vi "NXT_HINDBRAIN NXT Buttons To String.vi"(1 "_NXTButtonStates":bool[](array[boolean])) -> (0 "String":string)   [LabVIEW 2012, in "Tugboat.lvrbt"]
uses:
  Tugboat.lvrbt
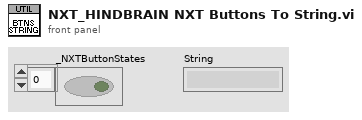
[diagram p1: front panel]
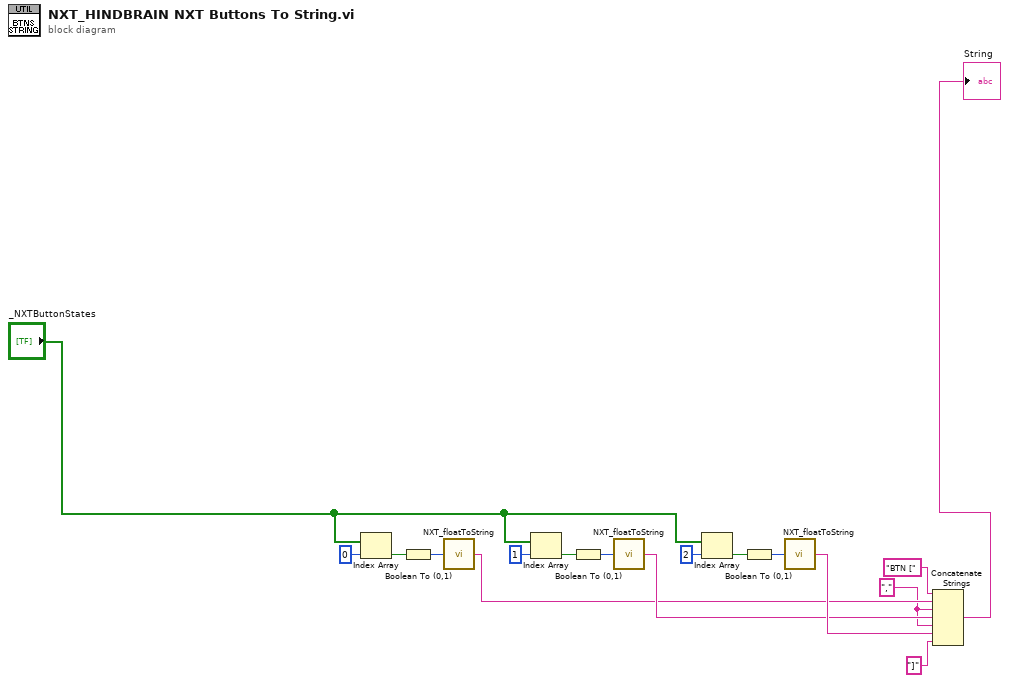
[diagram p0: block diagram]
diagram:
  w12 = "," ("string")
  n1 = Index Array(array="_NXTButtonStates", index=0) -> (element=w1:bool)
  n2 = Boolean To (0,1)(Boolean=w1) -> (0, 1=w3:i16)
  n3 = call <vilib>:"NXT_floatToString.vi"("number"=w3) -> ("string"=w14:string)
  n4 = Index Array(array="_NXTButtonStates", index=1) -> (element=w4:bool)
  n5 = Boolean To (0,1)(Boolean=w4) -> (0, 1=w6:i16)
  n6 = call <vilib>:"NXT_floatToString.vi"("number"=w6) -> ("string"=w15:string)
  n7 = Index Array(array="_NXTButtonStates", index=2) -> (element=w7:bool)
  n8 = Boolean To (0,1)(Boolean=w7) -> (0, 1=w9:i16)
  n9 = call <vilib>:"NXT_floatToString.vi"("number"=w9) -> ("string"=w16:string)
  n10 = Concatenate Strings("BTN [" ("string"), w14, w12, w15, w12, w16, "]" ("string")) -> (→"String":string)
